vi "JSON Edit.vi"(4 "Enums as string? (F)":bool, 6 "Pretty Print? (F)":bool, 7 "Variant in":variant, 8 "error in (no error)":errorcluster, 9 "Action (Get or Create)":T1, 10 "Root Path ([]=Root)":string[](array[string]), 11 "JSON in":string) -> (0 "error out":errorcluster, 1 "Exists?":bool, 2 "JSON out":string, 3 "Variant out":variant)   [LabVIEW 2019, in "labview_json.lvlib"]
doc: "Edit the <b>JSON in</b> string to create, get, set or delete elements by the <b>Variant in</b>. \n<b>Actions</b>:\n <b>Get or Create</b> - Get or create variant elements if necessary.\n <b>Get</b> - Get variant elements only.\n <b>Set</b> - Set or create variant elements if necessary.\n <b>Pop</b> - Get and delete variant elements if exists.\nSpecify the <b>Root Path</b> to the nested object key or array index. \n<b>Exists?</b> only returns True if all elements are found. \n<b>Pretty Print?</b> whitespace indents the <b>JSON out</b> string.\nCreated by: Ryan Pacini"
uses:
  labview_json.lvlib
  JSON Action.ctl
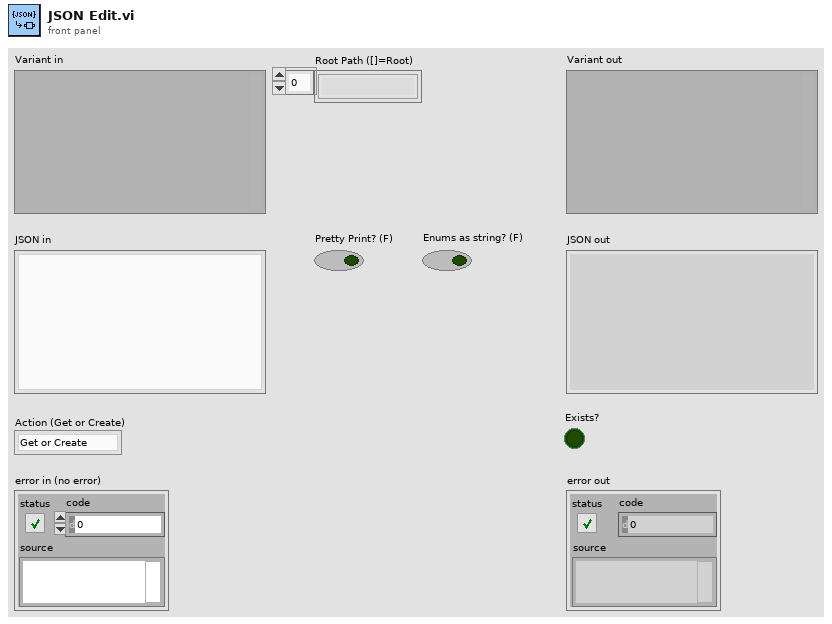
[diagram p1: front panel]
types:
  T1 = typedef "labview_json.lvlib/JSON Action.ctl" = enum8{"Get or Create", "Get", "Set"}
  T2 = typedef "labview_json.lvlib/Element.ctl" = cluster{"Key":string, "Type":T3, "Value":variant}
  T3 = typedef "labview_json.lvlib/Element Type.ctl" = enum8{"NULL", "BOOL", "INT", "UINT", "FLOAT", "STRING", "ARRAY", "OBJECT", "SKIP"}
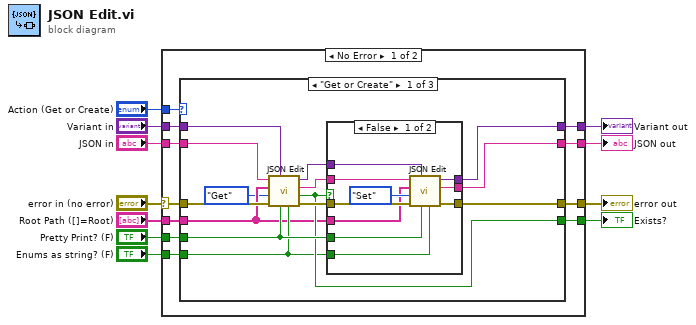
[diagram p0: block diagram]
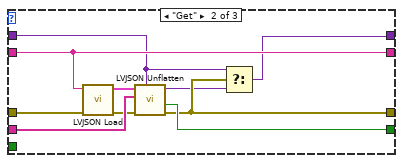
[diagram p3: hidden frame]
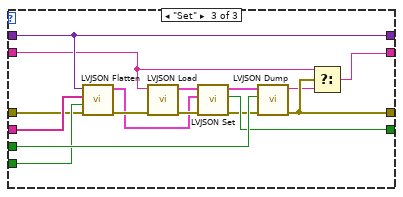
[diagram p4: hidden frame]
diagram:
  n1 = case shown="No Error" "error in (no error)" {
    selector: "error in (no error)" -> [w22 w78]
    tunnel: [w21 w78] -> w10
    tunnel: "JSON in" -> [w20 w77]
    tunnel: [w19 w77] -> w8
    tunnel: "Root Path ([]=Root)" -> [w18 _]
    tunnel: "Variant in" -> [w15 w76]
    tunnel: "Pretty Print? (F)" -> [w17 _]
    tunnel: [w16 _] -> w4
    tunnel: "Action (Get or Create)" -> [w14 _]
    tunnel: [w13 w76] -> w2
    tunnel: "Enums as string? (F)" -> [w12 _]
    frame No Error {
      n2 = case shown="\"Get or Create\"" w14 {
        tunnel: w22 -> [w33 w59 w68]
        tunnel: [w36 w52 w63] -> w21
        tunnel: w20 -> [w26 w57 w62]
        tunnel: [w35 w57 w60] -> w19
        tunnel: w18 -> [w25 w56 w69]
        tunnel: w17 -> [w32 _ w75]
        tunnel: [w30 w58 w74] -> w16
        tunnel: w15 -> [w24 w53 w71]
        tunnel: [w34 w50 w71] -> w13
        tunnel: w12 -> [w27 _ w70]
        frame "Get or Create" {
          n3 = call "JSON Edit.vi"("Enums as string? (F)"=w27, "Pretty Print? (F)"=w32, "Variant in"=w24, "error in (no error)"=w33, "Action (Get or Create)"=JSON_Action."Get", "Root Path ([]=Root)"=w25, "JSON in"=w26) -> ("error out"=w31:errorcluster, "Exists?"=w30:bool, "JSON out"=w28:string, "Variant out"=w29:variant)  [unwired: 1 in]
          n4 = case shown="False" w30 {
            tunnel: w31 -> [w46 w48]
            tunnel: w32 -> [w42 _]
            tunnel: [w45 w48] -> w36
            tunnel: [w43 w49] -> w35
            tunnel: w29 -> [w37 w47]
            tunnel: [w44 w47] -> w34
            tunnel: w28 -> [w38 w49]
            tunnel: w25 -> [w39 _]
            tunnel: w27 -> [w41 _]
            frame False {
              n5 = call "JSON Edit.vi"("Enums as string? (F)"=w41, "Pretty Print? (F)"=w42, "Variant in"=w37, "error in (no error)"=w46, "Action (Get or Create)"=JSON_Action."Set", "Root Path ([]=Root)"=w39, "JSON in"=w38) -> ("error out"=w45:errorcluster, "JSON out"=w43:string, "Variant out"=w44:variant)  [unwired: 1 in, 1 out]
            }
            frame True {
              # "All keys found"
            }
          }
        }
        frame "Get" {
          n6 = call "LVJSON Load.vi"("error in (no error)"=w59, "JSON in"=w57) -> ("error out"=w55:errorcluster, "Root Element out"=w54:T2)  [unwired: 7 in, 1 out]
          n7 = call "LVJSON Unflatten.vi"("Variant Type"=w53, "error in (no error)"=w55, "Root Path ([]=Root)"=w56, "Root Element in"=w54) -> ("error out"=w52:errorcluster, "Exists?"=w58:bool, "Variant out"=w51:variant)  [unwired: 4 in, 1 out]
          n8 = Select(t=w53, s=w52, f=w51) -> (s? t:f=w50:variant)
        }
        frame "Set" {
          n9 = call "LVJSON Flatten.vi"("error in (no error)"=w68, "Enums as string? (F)"=w70, "Root Path ([]=Root)"=w69, "Variant in"=w71) -> ("error out"=w67:errorcluster, "Root Element out"=w64:T2)  [unwired: 6 in]
          n10 = call "LVJSON Load.vi"("error in (no error)"=w67, "JSON in"=w62) -> ("error out"=w65:errorcluster, "Root Element out"=w66:T2)  [unwired: 7 in, 1 out]
          n11 = call "LVJSON Set.vi"("error in (no error)"=w65, "Root Element to Merge"=w64, "Root Element in"=w66) -> ("error out"=w72:errorcluster, "Exists?"=w74:bool, "Root Element out"=w73:T2)  [unwired: 6 in]
          n12 = call "LVJSON Dump.vi"("error in (no error)"=w72, "Pretty Print? (F)"=w75, "Root Element in"=w73) -> ("error out"=w63:errorcluster, "JSON out"=w61:string)  [unwired: 6 in, 1 out]
          n13 = Select(t=w62, s=w63, f=w61) -> (s? t:f=w60:string)
        }
      }
    }
    frame Error {
    }
  }
  "error out" <- w10
  "JSON out" <- w8
  "Exists?" <- w4
  "Variant out" <- w2
